vi "Get XY Plot Properties from Variant.vi"(6 "Plot#":i32, 8 "error in (no error)":errorcluster, 11 "variant":variant) -> (0 "error out":errorcluster, 2 "Plot":T1, 3 "variant dup":variant)   [LabVIEW 2020, in "Workspace MultiY Graph.lvlib"]
uses:
  Workspace MultiY Graph.lvlib
  XY Plot Properties.ctl
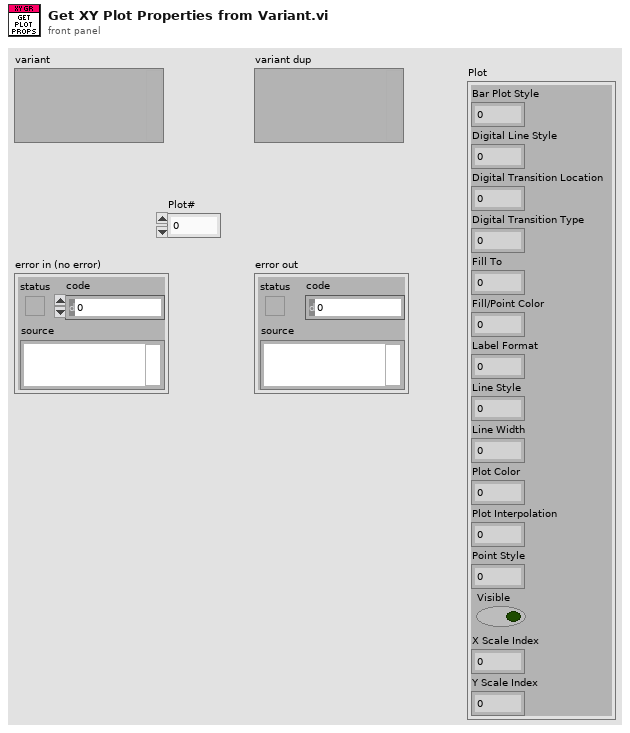
[diagram p1: front panel]
types:
  T1 = typedef "Workspace MultiY Graph.lvlib/XY Plot Properties.ctl" = cluster{"Bar Plot Style":u8, "Digital Line Style":u8, "Digital Transition Location":u8, "Digital Transition Type":u8, "Fill To":i16, "Fill/Point Color":u32, "Label Format":u8, "Line Style":u8, "Line Width":u8, "Plot Color":u32, "Plot Interpolation":u8, "Point Style":u8, "Visible":bool, "X Scale Index":u32, "Y Scale Index":u32}
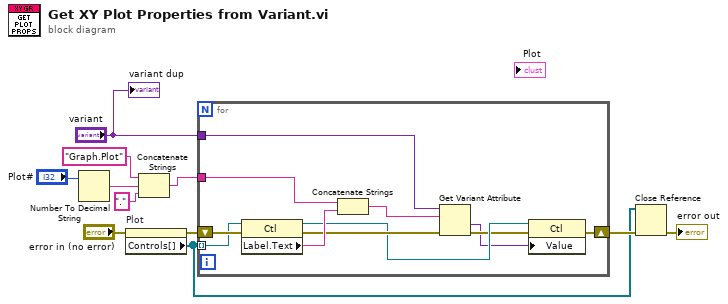
[diagram p0: block diagram]
diagram:
  n1 = Number To Decimal String(number="Plot#") -> (decimal integer string=w3:string)  [unwired: 1 in]
  n2 = property on="Plot" class="Clust (strict)"(error in="error in (no error)") -> (error out=w10:errorcluster, "Controls[]"=w8:refnum<vi>[])  [unwired: 1 in, 1 out]
  n3 = Concatenate Strings("Graph.Plot" ("name"), w3, "." ("string")) -> (w2:string)
  n4 = for {
    tunnel: w8 -> [w21] mode=indexing
    tunnel: w2 -> [w19]
    shift-right: [w20] -> w9
    shift-left: w10 -> [w22]
    tunnel: "variant" -> [w18]
    n5 = property on="Property Node" class="Ctl"(reference=w21, error in=w22) -> (reference out=w14:refnum<vi>, error out=w16:errorcluster, "Label.Text"=w17:string)
    n6 = Concatenate Strings(w19, w17) -> (w15:string)
    n7 = Get Variant Attribute(Variant=w18, name=w15, error in=w16) -> (value=w12:variant, error out=w13:errorcluster)  [unwired: 1 in, 2 out]
    n8 = property on="Property Node" class="Ctl"(reference=w14, error in=w13, "Value"=w12) -> (error out=w20:errorcluster)  [unwired: 1 out]
  }
  n9 = Close Reference(reference=w8, error in (no error)=w9) -> (error out=→"error out":errorcluster)
  "variant dup" <- "variant"
